vi "ProcessStop.vi"(9 "Cluster in":T1, 11 "Cluster":T2) -> (1 "Cluster out":T1, 3 "output cluster":T2)   [LabVIEW 2013]
uses:
  Control/SystemProcess.ctl
  Control/Buffer.vi
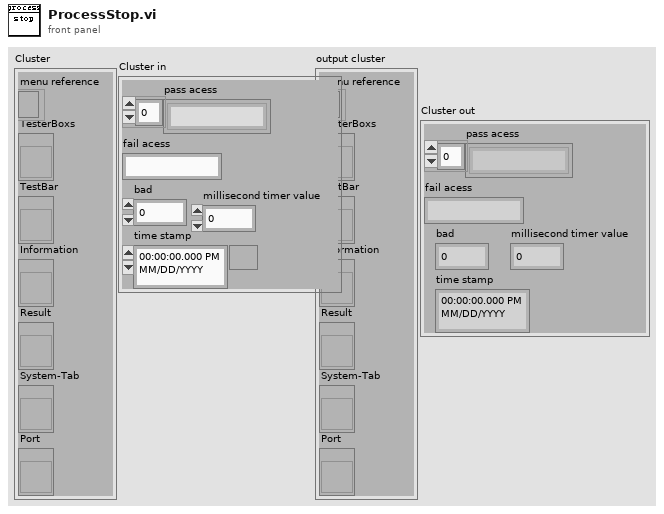
[diagram p1: front panel]
types:
  T1 = cluster{"pass acess":string[], "fail acess":string, "bad":i32, "time stamp":timestamp, "millisecond timer value":u32}
  T2 = cluster{"menu reference":refnum<k9>, "TesterBoxs":refnum<vi>, "TestBar":refnum<vi>, "Information":refnum<vi>, "Result":refnum<vi>, "System-Tab":refnum<vi>, "Port":refnum<vi>}
  T3 = typedef "SystemProcess.ctl" = enum16{"Idle", "SystemInit", "SpecialEvent", "Barcode(SN)", "TestInitialize", "Test", "Stop", "SaveTestData", "Exit"}
  T4 = typedef "StatusInformation.ctl" = cluster{"FileName:":string, "Barcode(S/N):":string, "TestStep:":string, "TestTime:":string, "Station:":string, "Model:":string, "Line:":string, "Status:":string, "Series:":string, "Reserve:":string}
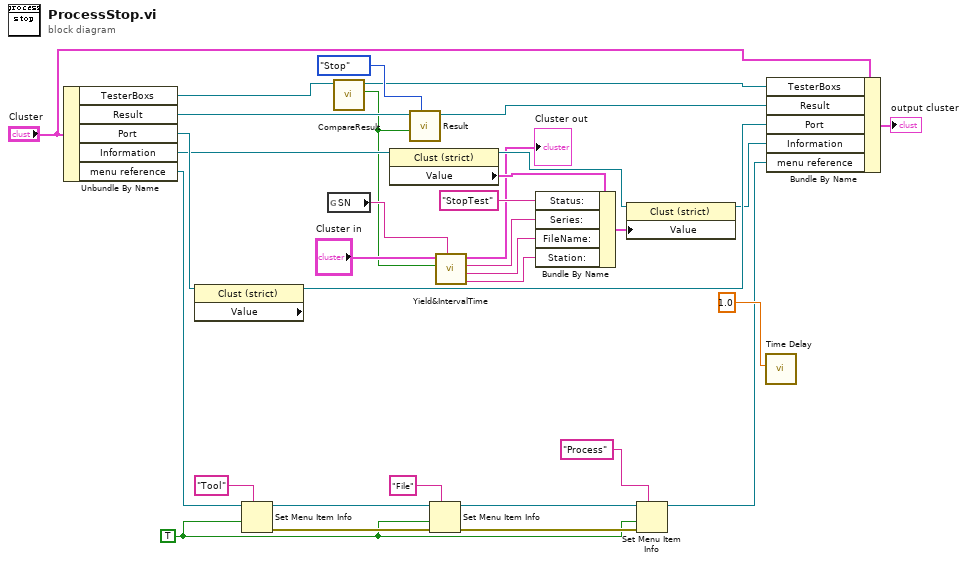
[diagram p0: block diagram]
diagram:
  w9 = TRUE ("enabled")
  n1 = Unbundle By Name("Cluster") -> ("TesterBoxs"=w29:refnum<vi>, "Result"=w32:refnum<vi>, "Port"=w27:refnum<vi>, "Information"=w26:refnum<vi>, "menu reference"=w16:refnum<k9>)
  n2 = property class="Clust (strict)" props=["Value"](reference=w27) -> (reference out=w28:refnum<vi>)  [unwired: 1 in, 2 out]
  n3 = Set Menu Item Info(7:"Tool" ("item tag"), 9:w9, 11:w16) -> (0:w18:errorcluster, 3:w19:refnum<k9>)  [unwired: 4 in]
  n4 = global read "Buffer.vi" "SN"() -> (w5:string)
  n5 = call "CompareResult.vi"("MulticolumnListbox in"=w29) -> ("Result"=w4:bool, "MulticolumnListbox out"=w30:refnum<vi>)  [unwired: 9 in]
  n6 = property class="Clust (strict)"(reference=w26) -> (reference out=w25:refnum<vi>, "Value"=w23:T4)  [unwired: 1 in, 1 out]
  n7 = call "Result.vi"("MainProcess"=SystemProcess."Stop", 9:"Result"=w4, 11:"Result"=w32) -> ("Result"=w33:refnum<vi>)  [unwired: 8 in]
  n8 = Set Menu Item Info(7:"File" ("item tag"), 8:w18, 9:w9, 11:w19) -> (0:w12:errorcluster, 3:w11:refnum<k9>)  [unwired: 3 in]
  n9 = call "Yield&IntervalTime.vi"("barcode"=w5, "result"=w4, "Cluster in"="Cluster in") -> ("fail"=w1:string, "pass"=w2:string, "Yield"=w3:string, "Cluster out"=→"Cluster out":T1)  [unwired: 5 in]
  n10 = Bundle By Name(cluster=w23, "Status:"="StopTest", "Series:"=w3, "FileName:"=w2, "Station:"=w1) -> (w22:T4)
  n11 = property class="Clust (strict)"(reference=w25, "Value"=w22) -> (reference out=w24:refnum<vi>)  [unwired: 1 in, 1 out]
  n12 = Set Menu Item Info(7:"Process" ("item name"), 8:w12, 9:w9, 11:w11) -> (3:w10:refnum<k9>)  [unwired: 3 in, 1 out]
  n13 = call "Time Delay"("Delay Time (s)"=1.0) -> ()  [unwired: 10 in, 1 out]
  n14 = Bundle By Name(cluster="Cluster", "TesterBoxs"=w30, "Result"=w33, "Port"=w28, "Information"=w24, "menu reference"=w10) -> (→"output cluster":T2)
